vi "Delete Record Assert Error.vi"(7 "Bulk Delete?":bool, 8 "Error In":errorcluster, 9 "Records":refnum<class "Expenses Tracker Record.lvclass">[](array[class]), 10 "Assertion Label":string, 11 "SQLite DB Operator In":refnum<class "SQLite DB Operator.lvclass">) -> (0 "Error Out":errorcluster, 3 "SQLite DB Operator Out":refnum<class "SQLite DB Operator.lvclass">)   [LabVIEW 2023]
uses:
  Clasess/SQLite DB Operator/SQLite DB Operator.lvclass
  Interfaces/Expenses Tracker Record/Expenses Tracker Record.lvclass
  <vilib>/addons/_JKI Toolkits/Caraya/classes/Assert/Assert Error.vi
  <vilib>/addons/_JKI Toolkits/Caraya/classes/Assert/Assert.lvclass
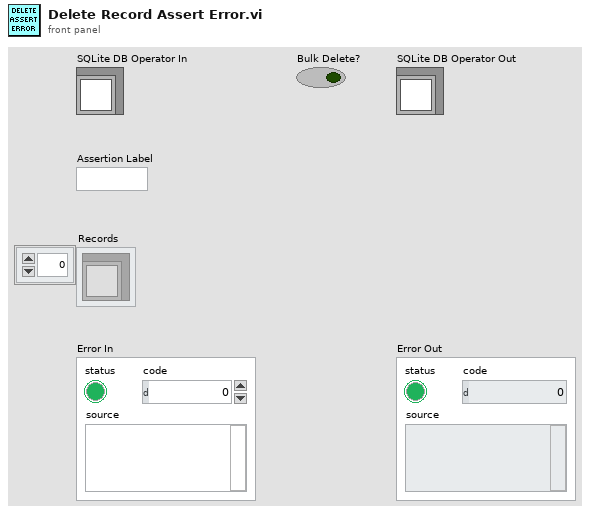
[diagram p1: front panel]
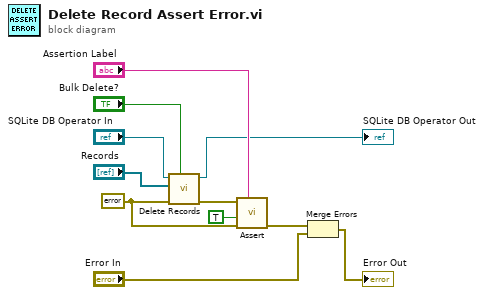
[diagram p0: block diagram]
diagram:
  w5 = errorcluster {"status"=FALSE, "code"=0, "source"=""} ("error in (no error)")
  n1 = call-dynamic "Delete Records.vi"("Bulk Delete?"="Bulk Delete?", "Error In (no error)"=w5, "Expenses Tracker Records In"="Records", "SQLite DB Operator In"="SQLite DB Operator In") -> ("Error Out"=w7:errorcluster, "SQLite DB Operator Out"=→"SQLite DB Operator Out":refnum<class "SQLite DB Operator.lvclass">)  [unwired: 5 in, 1 out]
  n2 = call-poly <vilib>:"Assert.vi"("Label"="Assertion Label", "error in (no error)"=w5, "Register with caller test (F)"=TRUE, "Error?"=w7) -> ("error out"=w11:errorcluster)  [unwired: 6 in, 1 out]
  n3 = Merge Errors(w11, "Error In") -> (→"Error Out":errorcluster)
